vi "DAQ Close.vi"(8 "error in (no error)":errorcluster caption="错误输入（无错误）", 11 "DAQ Tasks":T1 caption="DAQ任务") -> (0 "error out":errorcluster caption="错误输出")   [LabVIEW 2013]
uses:
  controls/DAQ Tasks.ctl
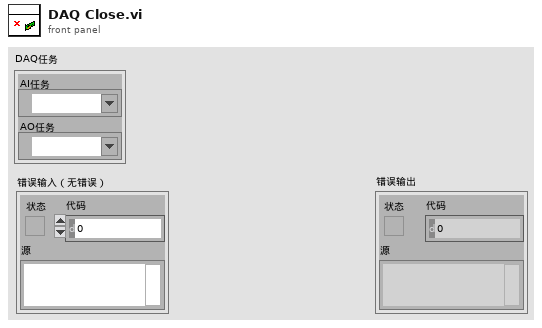
[diagram p1: front panel]
types:
  T1 = typedef "DAQ Tasks.ctl" = cluster{"AI Task":refnum<k21>, "AO Task":refnum<k21>}
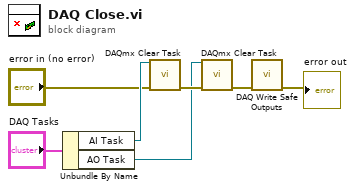
[diagram p0: block diagram]
diagram:
  n1 = Unbundle By Name("DAQ Tasks") -> ("AI Task"=w5:refnum<k21>, "AO Task"=w4:refnum<k21>)
  n2 = call <vilib>:"DAQmx Clear Task.vi"("task in"=w5, "error in"="error in (no error)") -> ("error out"=w6:errorcluster)  [unwired: 13 in]
  n3 = call <vilib>:"DAQmx Clear Task.vi"("task in"=w4, "error in"=w6) -> ("error out"=w2:errorcluster)  [unwired: 13 in]
  n4 = call "DAQ Write Safe Outputs.vi"("error in (no error)"=w2) -> ("error out"=→"error out":errorcluster)  [unwired: 10 in]
